vi "Device Code Write.vi"(4 "error in (no error)":errorcluster, 5 "Value":u32, 6 "Container State":T3, 7 "Display State In":T1={"Title"="", "Explanation"="", "Mode"=enum."myRIO-1900"}) -> (0 "error out":errorcluster, 3 "Display State Out":T1={"Title"="", "Explanation"="", "Mode"=enum."myRIO-1900"})   [LabVIEW 2021, in "myRIO Device Button.xctl"]
uses:
  <vilib>/myRIO/Common/Instrument Driver Framework/Utilities/xctls/myRIO Device Button/myRIO Device Button.xctl
  <vilib>/_xctls/Container State.ctl
  <vilib>/myRIO/Common/Instrument Driver Framework/Utilities/xctls/myRIO Device Button/State.ctl
  <vilib>/myRIO/Common/Instrument Driver Framework/Utilities/typedefs/Hardware Version Enum.ctl
  <vilib>/_xctls/XControlSupport.lvlib
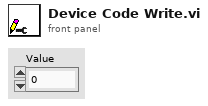
[diagram p1: front panel]
types:
  T1 = typedef "myRIO Device Button.xctl/State.ctl" = cluster{"Title":string, "Explanation":string, "Mode":T2}
  T2 = typedef "Hardware Version Enum.ctl" = enum16{"Unknown", "myRIO-1900", "myRIO-1950", "roboRIO", "NI ELVIS RIO CM", "ELVIS III"}
  T3 = typedef "XControlSupport.lvlib/Container State.ctl" = cluster{"Indicator?":bool, "Run Mode?":bool, " Refnum":refnum<vi>}
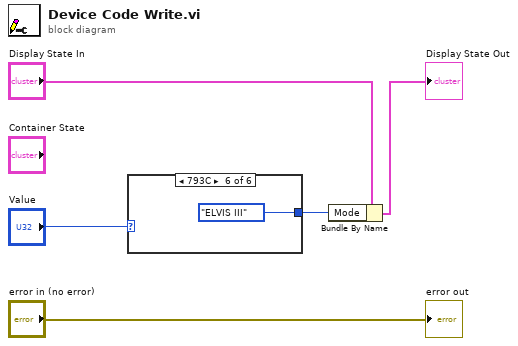
[diagram p0: block diagram]
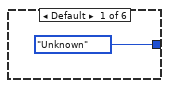
[diagram p2: hidden frame]
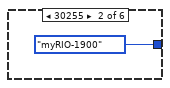
[diagram p3: hidden frame]
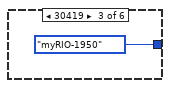
[diagram p4: hidden frame]
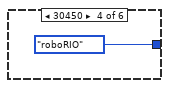
[diagram p5: hidden frame]
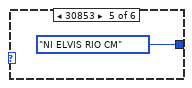
[diagram p6: hidden frame]
diagram:
  n1 = case shown="793C" "Value" {
    tunnel: [Hardware_Version_Enum."Unknown" ("Mode") Hardware_Version_Enum."myRIO-1900" ("Mode") Hardware_Version_Enum."myRIO-1950" ("Mode") Hardware_Version_Enum."roboRIO" ("Mode") Hardware_Version_Enum."NI ELVIS RIO CM" ("Mode") Hardware_Version_Enum."ELVIS III" ("Mode")] -> w3
    frame Default {
    }
    frame 30255 {
    }
    frame 30419 {
    }
    frame 30450 {
    }
    frame 30853 {
    }
    frame 31036 {
    }
  }
  n2 = Bundle By Name(cluster="Display State In", "Mode"=w3) -> (→"Display State Out":T1)
  "error out" <- "error in (no error)"
